vi "Delete Blob.vi"(8 "error in (no error)":errorcluster, 9 "Blob":string, 10 "Container":string, 11 "Azure Session in":refnum<class "Session.lvclass">) -> (0 "error out":errorcluster, 3 "Azure Session out":refnum<class "Session.lvclass">)   [LabVIEW 2015, in "NI_Azure_Blob.lvlib"]
doc: "Marks a blob for deletion."
uses:
  NI_Azure_Blob.lvlib
  Core/Session/Session.lvclass
  Core/Name Value Pair.ctl
  Core/Session/Session.lvclass/Session.ctl
  Core/Session/Write HTTP Verb.vi
  Core/Session/Write URL Suffix.vi
  Core/Session/Write Request Headers.vi
  Core/NI_Azure_Core.lvlib
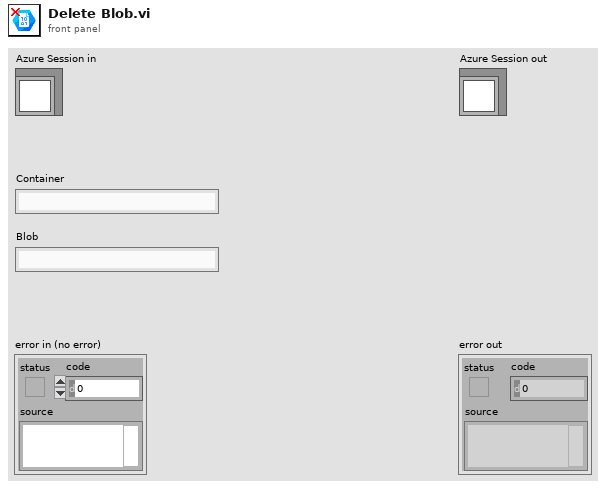
[diagram p1: front panel]
types:
  T1 = typedef "NI_Azure_Core.lvlib/Name Value Pair.ctl" = cluster{"name":string, "value":string}
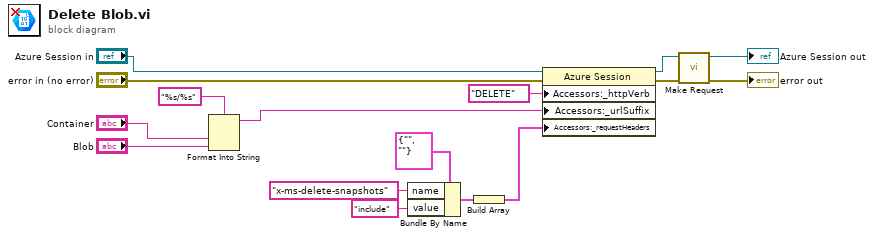
[diagram p0: block diagram]
diagram:
  n1 = Format Into String(format string="%s/%s", "Container", "Blob") -> (resulting string=w6:string)  [unwired: 2 in, 1 out]
  n2 = Bundle By Name(cluster=T1 {"name"="", "value"=""} ("Name Value Pair"), "name"="x-ms-delete-snapshots", "value"="include") -> (w2:T1)
  n3 = Build Array(w2) -> (w1:T1[])
  n4 = property class="Azure Session"(reference="Azure Session in", error in="error in (no error)", "Accessors:_httpVerb"="DELETE" ("HTTP-Verb"), "Accessors:_urlSuffix"=w6, "Accessors:_requestHeaders"=w1) -> (reference out=w8:refnum<class "Session.lvclass">, error out=w10:errorcluster)
  n5 = call "Make Request.vi"("error in (no error)"=w10, "Session in"=w8) -> ("error out"=→"error out":errorcluster, "Session out"=→"Azure Session out":refnum<class "Session.lvclass">)  [unwired: 7 in, 1 out]
